vi "Chronos TDMS Read Channel Data as XY.vi"(8 "error in (no error)":errorcluster, 10 "Files":path[](array[path]), 11 "Limit Plot Map":T1) -> (0 "error out":errorcluster, 1 "Current File":T4, 3 "Plot Map out":T1)   [LabVIEW 2021]
uses:
  typedefs/Chronos cluster Current File.ctl
  GUI/Chronos cluster Map Limit Plots.ctl
  typedefs/Chronos cluster Plot Data and Limits.ctl
  Viewer/cluster CC Channel from TDMS.ctl
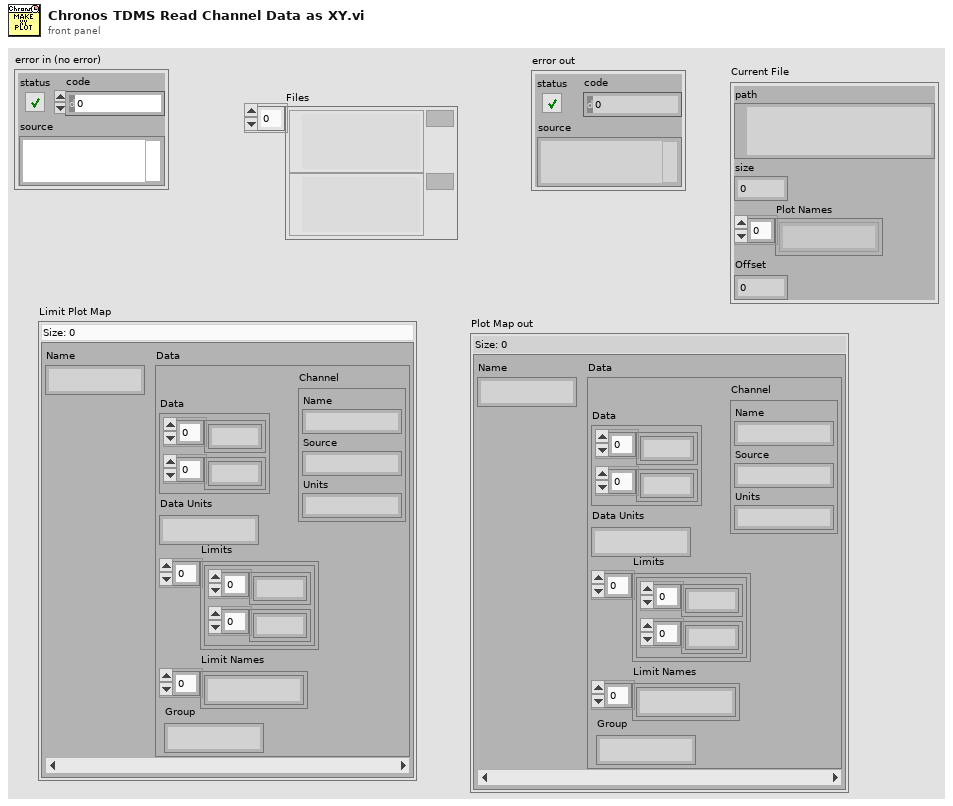
[diagram p1: front panel]
types:
  T1 = typedef "Chronos cluster Map Limit Plots.ctl" = map{string, T2}
  T2 = typedef "Chronos cluster Plot Data and Limits.ctl" = cluster{"Data":cluster{dbl[], dbl[]}, "Data Units":string, "Limits":cluster{dbl[], dbl[]}[], "Limit Names":string[], "Channel":T3, "Group":string}
  T3 = typedef "cluster CC Channel from TDMS.ctl" = cluster{"Name":string, "Source":string, "Units":string}
  T4 = typedef "Chronos cluster Current File.ctl" = cluster{"path":path, "size":i64, "Plot Names":string[], "Offset":i32}
  T5 = enum16{"open", "open or create", "create or replace", "create", "open (read-only)"}
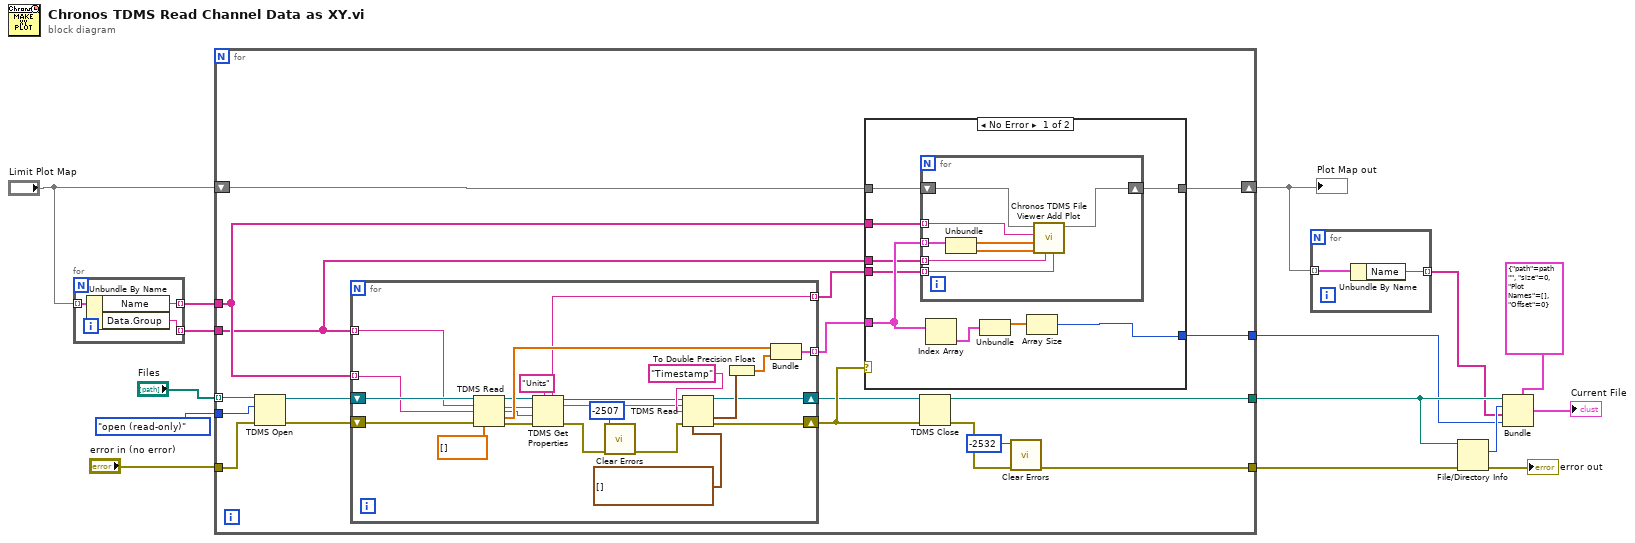
[diagram p0: block diagram]
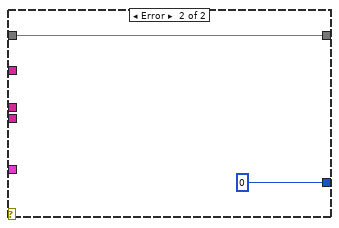
[diagram p2: hidden frame]
diagram:
  n1 = for {
    tunnel: "Limit Plot Map" -> [w18] mode=indexing
    tunnel: [w17] -> w3 mode=indexing
    tunnel: [w16] -> w1 mode=indexing
    n2 = Unbundle By Name(w18) -> ("Name"=w17:string, "Data.Group"=w16:string)
  }
  n3 = for {
    tunnel: "Files" -> [w29] mode=indexing
    tunnel: T5."open (read-only)" ("operation (0:open)") -> [w34]
    tunnel: [w31] -> w12
    tunnel: [w30] -> w2
    tunnel: "error in (no error)" -> [w33]
    tunnel: [w23] -> w8
    shift-right: [w27] -> w6
    shift-left: "Limit Plot Map" -> [w28]
    tunnel: w3 -> [w26]
    tunnel: w1 -> [w20]
    n4 = TDMS Open(8:w33, 10:w34, 11:w29) -> (0:w36:errorcluster, 3:w35:refnum<k34>)  [unwired: 4 in]
    n5 = for {
      tunnel: w26 -> [w47] mode=indexing
      shift-right: [w38] -> w25
      shift-left: w36 -> [w60]
      shift-right: [w37] -> w24
      shift-left: w35 -> [w59]
      tunnel: w20 -> [w48] mode=indexing
      tunnel: [w52] -> w21 mode=indexing
      tunnel: [w50] -> w19 mode=indexing
      w51 = "Units" ("property name")
      n6 = TDMS Read(0:w59, 5:w48, 7:w47, 11:w60, 12:dbl[] []) -> (4:w46:refnum<k34>, 6:w44:string, 8:w43:string, 10:w53:dbl[], 15:w45:errorcluster)  [unwired: 3 in, 1 out]
      n7 = TDMS Get Properties(5:w51, 7:w51, 8:w45, 9:w43, 10:w44, 11:w46) -> (0:w40:errorcluster, 2:w41:string, 3:w42:refnum<k34>, 4:w50:string)  [unwired: 2 out]
      n8 = call <vilib>:"Clear Errors.vi"("error in (no error)"=w40, "specific error code to clear (0: all)"=-2507) -> ("error out"=w39:errorcluster)  [unwired: 4 in, 1 out]
      n9 = TDMS Read(0:w42, 5:w41, 7:"Timestamp", 11:w39, 12:timestamp[] []) -> (4:w37:refnum<k34>, 10:w55:timestamp[], 15:w38:errorcluster)  [unwired: 3 in, 3 out]
      n10 = To Double Precision Float(number=w55) -> (double precision float=w54:dbl[])
      n11 = Bundle(w53, w54) -> (w52:cluster{dbl[], dbl[]})  [unwired: 1 in]
    }
    n12 = case shown="No Error" w25 {
      tunnel: w21 -> [w64 _]
      tunnel: [w63 0] -> w30
      tunnel: w26 -> [w69 _]
      tunnel: w28 -> [w68 w78]
      tunnel: [w67 w78] -> w27
      tunnel: w20 -> [w62 _]
      tunnel: w19 -> [w61 _]
      frame No Error {
        n13 = for {
          tunnel: w64 -> [w74] mode=indexing
          tunnel: w69 -> [w76] mode=indexing
          shift-right: [w75] -> w67
          shift-left: w68 -> [w77]
          tunnel: w62 -> [w71] mode=indexing
          tunnel: w61 -> [w70] mode=indexing
          n14 = Unbundle(w74) -> (w73:dbl[], w72:dbl[])
          n15 = call "Chronos TDMS File Viewer Add Plot.vi"("Data Units"=w70, "Group"=w71, "Times"=w72, "Data"=w73, "Name"=w76, "Limit Plot Map"=w77) -> ("Plot Map out"=w75:T1)  [unwired: 5 in]
        }
        n16 = Index Array(array=w64) -> (element=w65:cluster{dbl[], dbl[]})  [unwired: 1 in]
        n17 = Unbundle(w65) -> (w66:dbl[])  [unwired: 1 out]
        n18 = Array Size(array=w66) -> (size(s)=w63:i32)
      }
      frame Error {
      }
    }
    n19 = TDMS Close(8:w25, 11:w24) -> (0:w32:errorcluster, 3:w31:path)
    n20 = call <vilib>:"Clear Errors.vi"("error in (no error)"=w32, "specific error code to clear (0: all)"=-2532) -> ("error out"=w23:errorcluster)  [unwired: 4 in, 1 out]
  }
  "Plot Map out" <- w6
  n21 = for {
    tunnel: [w80] -> w5 mode=indexing
    tunnel: w6 -> [w81] mode=indexing
    n22 = Unbundle By Name(w81) -> ("Name"=w80:string)
  }
  n23 = File/Directory Info(path=w12, error in=w8) -> (size=w10:i64, error out=→"error out":errorcluster)  [unwired: 5 out]
  n24 = Bundle(cluster=T4 {"path"=path "", "size"=0, "Plot Names"=[], "Offset"=0} ("Current File"), "path"=w12, "size"=w10, "Plot Names"=w5, "Offset"=w2) -> (→"Current File":T4)
